vi "LeCroy Wave Series Acquire Multiple Waveforms.vi"() -> ()   [LabVIEW 2013]
doc: "This example shows how to configure multiple channels and acquire waveforms from multiple channels."
uses:
  <instrlib>/LeCroy Wave Series/Public/Configure/Configure Edge Trigger.vi
  <instrlib>/LeCroy Wave Series/Public/Data/Read Multiple Waveforms.vi
  <instrlib>/LeCroy Wave Series/LeCroy Wave Series.lvlib
panel:
  in  "Channel (1: Channel 2)":u16(ring)=2 items=["Channel 1", "Channel 2", "Channel 3", "Channel 4"]
  in  "Channel (0: Channel 1)":u16(ring)=1 items=["Channel 1", "Channel 2", "Channel 3", "Channel 4"]
  in  "Vertical Coupling (0: A1M)":u16(ring) items=["A1M", "D1M", "D50", "Ground"]
  in  "Vertical Coupling (0: A1M)":u16(ring) items=["A1M", "D1M", "D50", "Ground"]
  in  "Vertical Offset (0.0 V)":dbl
  in  "Vertical Offset (0.0 V)":dbl
  in  "Probe Attenuation (-1)":dbl=-1.0
  in  "Probe Attenuation (-1)":dbl=-1.0
  in  "Timeout (10000 ms)":u32=10000
  out "Waveform Data":waveform(dbl)[](graph)
  in  "VISA resource name":refnum<visa-resource-name>="VICP::169.254.20.90"
  # "(c) 2005 - 2012 NATIONAL INSTRUMENTS.  ALL RIGHTS RESERVED."
  # "Channel A"
  # "Channel B"
  # "Note:\nThis VI will time out without acquiring any data if the input signal on channel 1 does not cross 0 V trigger level with positive slope.\nFor more details on triggering pleas see the Edge Triggered Acquisition Example VI."
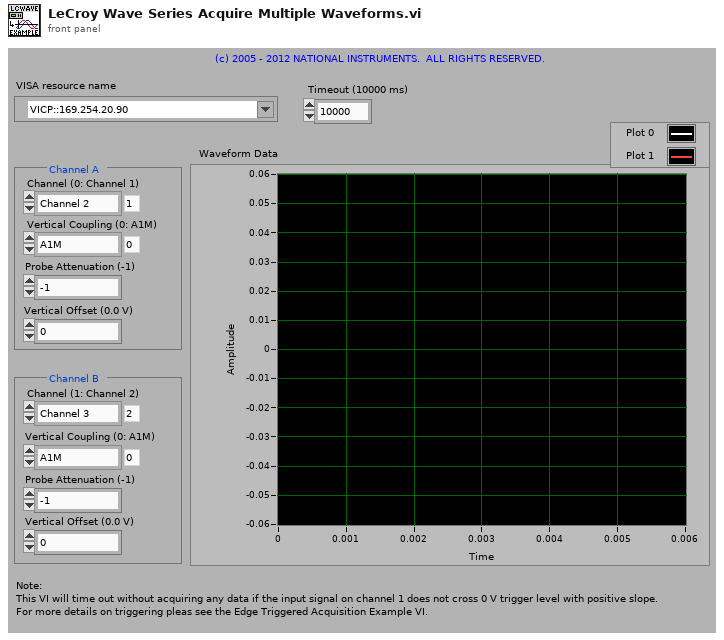
[diagram p1: front panel]
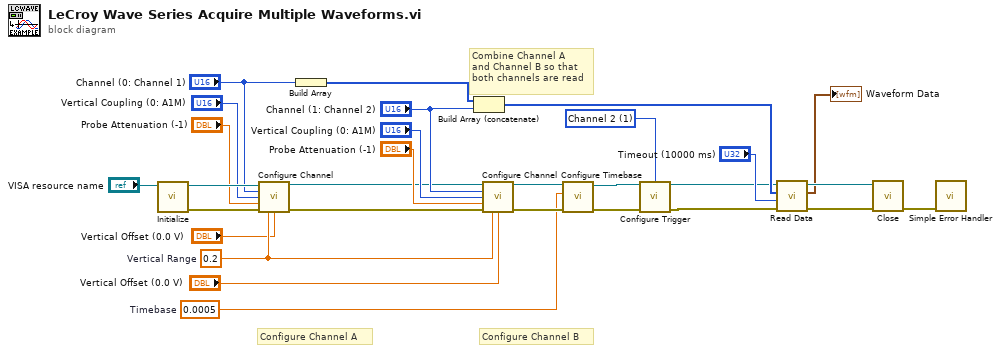
[diagram p0: block diagram]
diagram:
  w1 = u16 1 items=["Channel 1", "Channel 2", "Channel 3", "Channel 4", "External", "Line", "Ext", "Ext10"] ("Trigger Source (0: Channel 1)")
  w19 = 0.2  # Vertical Range
  w18 = 0.0005  # Timebase
  # "Combine Channel A\nand Channel B so that\nboth channels are read"
  # "Configure Channel B"
  # "Configure Channel A"
  n1 = call <instrlib>:"Initialize.vi"("VISA resource name"="VISA resource name") -> ("error out"=w24:errorcluster, "VISA resource name out"=w25:refnum<visa-resource-name>)  [unwired: 9 in]
  n2 = call <instrlib>:"Configure Channel.vi"("VISA resource name"=w25, "Channel (0: Channel 1)"="Channel (0: Channel 1)", "Vertical Coupling (0: A1M)"="Vertical Coupling (0: A1M)", "Probe Attenuation (-1.0)"="Probe Attenuation (-1)", "error in (no error)"=w24, "Vertical Range (10.0 V)"=w19, "Vertical Offset (0.0 V)"="Vertical Offset (0.0 V)") -> ("VISA resource name out"=w8:refnum<visa-resource-name>, "error out"=w7:errorcluster)  [unwired: 7 in]
  n3 = Build Array("Channel (0: Channel 1)") -> (w10:u16[])
  n4 = Build Array (concatenate)(w10, "Channel (1: Channel 2)") -> (w9:u16[])
  n5 = call <instrlib>:"Configure Channel.vi"("VISA resource name"=w8, "Channel (0: Channel 1)"="Channel (1: Channel 2)", "Vertical Coupling (0: A1M)"="Vertical Coupling (0: A1M)", "Probe Attenuation (-1.0)"="Probe Attenuation (-1)", "error in (no error)"=w7, "Vertical Range (10.0 V)"=w19, "Vertical Offset (0.0 V)"="Vertical Offset (0.0 V)") -> ("VISA resource name out"=w23:refnum<visa-resource-name>, "error out"=w22:errorcluster)  [unwired: 7 in]
  n6 = call <instrlib>:"Configure Timebase.vi"("error in (no error)"=w22, "Timebase (0.0005 s)"=w18, "VISA resource name"=w23) -> ("error out"=w5:errorcluster, "VISA resource name out"=w3:refnum<visa-resource-name>)  [unwired: 7 in]
  n7 = call-poly <instrlib>:"Configure Trigger.vi"("VISA resource name"=w3, "Trigger Source (0: Channel 1)"=w1, "error in (no error)"=w5) -> ("VISA resource name out"=w2:refnum<visa-resource-name>, "error out"=w4:errorcluster)  [unwired: 11 in]
  n8 = call-poly <instrlib>:"Read Data.vi"("error in (no error)"=w4, "Timeout (10000 ms)"="Timeout (10000 ms)", "Channels"=w9, "VISA resource name"=w2) -> ("error out"=w26:errorcluster, "Waveform Data"=→"Waveform Data":waveform(dbl)[], "VISA resource name out"=w27:refnum<visa-resource-name>)  [unwired: 5 in]
  n9 = call <instrlib>:"Close.vi"("error in (no error)"=w26, "VISA resource name"=w27) -> ("error out"=w28:errorcluster)  [unwired: 9 in]
  n10 = call <vilib>:"Simple Error Handler.vi"("error in (no error)"=w28) -> ()  [unwired: 4 in, 5 out]
